vi "Get All VIs in Memory.vi"(8 "error in (no error)":errorcluster, 11 "App Ref":refnum<vi>) -> (0 "error out":errorcluster, 2 "All VIs in Memory":string[](array[string]), 3 "App Ref out":refnum<vi>)   [LabVIEW 2020, in "MacroAssert.lvlib"]
doc: "Outputs all VIs in memory for <B>App Ref</B>."
uses:
  MacroAssert.lvlib
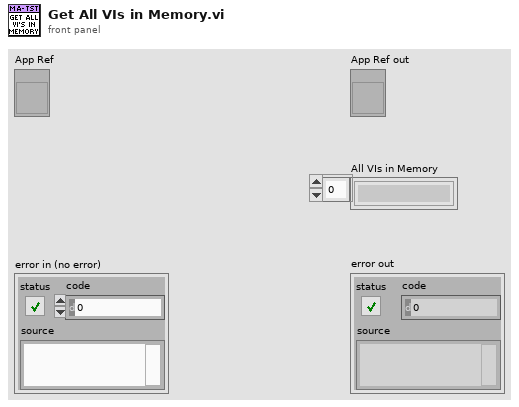
[diagram p1: front panel]
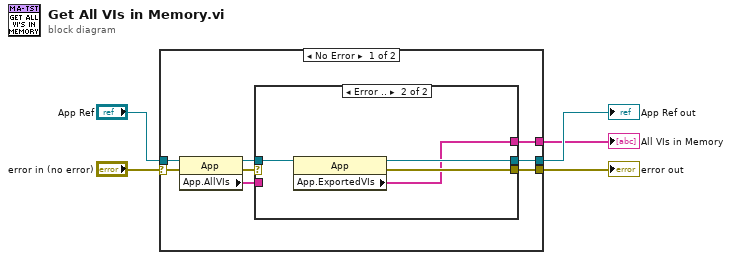
[diagram p0: block diagram]
diagram:
  n1 = case shown="No Error" "error in (no error)" {
    selector: "error in (no error)" -> [w12 w22]
    tunnel: [w11 w22] -> w4
    tunnel: "App Ref" -> [w10 w21]
    tunnel: [w8 w21] -> w2
    tunnel: [w6 _] -> w1
    frame No Error {
      n2 = property class="App"(reference=w10, error in=w12) -> (reference out=w9:refnum<vi>, error out=w13:errorcluster, "App.AllVIs"=w7:string[])
      n3 = case shown="Error .." w13 {
        selector: w13 -> [w16 _]
        tunnel: w9 -> [w15 w19]
        tunnel: [w16 w20] -> w11
        tunnel: [w15 w18] -> w8
        tunnel: w7 -> [w14 _]
        tunnel: [w14 w17] -> w6
        frame No Error {
        }
        frame Error {
          n4 = property class="App"(reference=w19) -> (reference out=w18:refnum<vi>, error out=w20:errorcluster, "App.ExportedVIs"=w17:string[])  [unwired: 1 in]
        }
      }
    }
    frame Error {
      # "If incoming error, just pass it through without doing anything"
    }
  }
  "App Ref out" <- w2
  "error out" <- w4
  "All VIs in Memory" <- w1
